vi "Read Map.vi"(8 "error in":errorcluster, 11 "Ballard ARINC-429 Rx Execution Unit in":refnum<class "Rx Execution Unit.lvclass">) -> (0 "error out":errorcluster, 2 "map":T1, 3 "Ballard ARINC-429 Rx Execution Unit out":refnum<class "Rx Execution Unit.lvclass">)   [LabVIEW 2020, in "AIM ARINC 429 Engine.lvlib" / "Implementation.lvlib" / "Rx Execution Unit.lvclass"]
uses:
  Rx Execution Unit.lvclass
  Shared/Map of Identifiers to Indexes.ctl
  Rx Execution Unit.lvclass/Rx Execution Unit.ctl
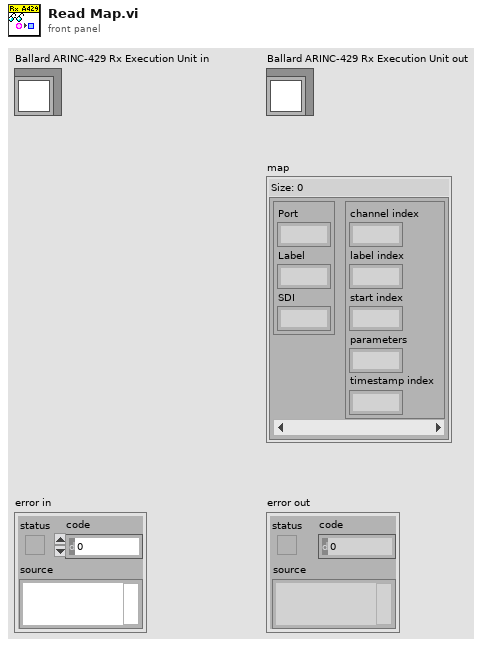
[diagram p1: front panel]
types:
  T1 = typedef "Map of Identifiers to Indexes.ctl" = map{cluster{"Port":u8, "Label":u8, "SDI":u8}, cluster{"channel index":i32, "label index":i32, "start index":i32, "parameters":i32, "timestamp index":i32}}
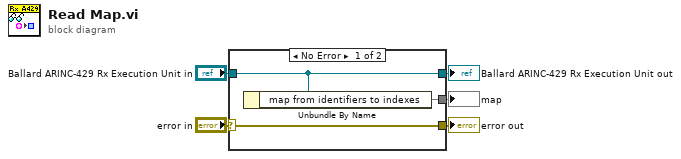
[diagram p0: block diagram]
diagram:
  n1 = case shown="No Error" "error in" {
    selector: "error in" -> [w8 w9]
    tunnel: [w8 w9] -> w4
    tunnel: [w7 w10] -> w2
    tunnel: "Ballard ARINC-429 Rx Execution Unit in" -> [w7 w10]
    tunnel: [w6 _] -> w1
    frame No Error {
      n2 = Unbundle By Name(w7) -> ("map from identifiers to indexes"=w6:T1)
    }
    frame Error {
    }
  }
  "error out" <- w4
  "Ballard ARINC-429 Rx Execution Unit out" <- w2
  "map" <- w1
